vi "Write CRDS.vi"(8 "error in (no error)":errorcluster, 10 "CRDS":refnum<class "CRDS Data.lvclass">, 11 "Nicholas Data in":refnum<class "Nicholas Data.lvclass">) -> (0 "error out":errorcluster, 3 "Nicholas Data out":refnum<class "Nicholas Data.lvclass">)   [LabVIEW 2014, in "Nicholas Data.lvclass"]
uses:
  Nicholas Data.lvclass
  Reusable/CRDS/Data/Main/CRDS Data.lvclass
  Nicholas Data.lvclass/Nicholas Data.ctl
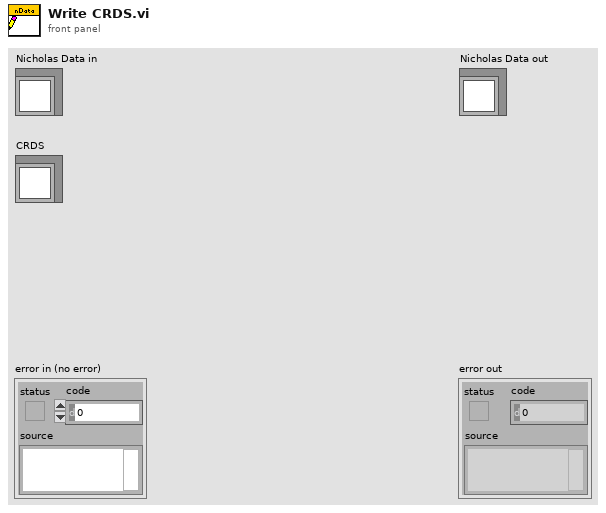
[diagram p1: front panel]
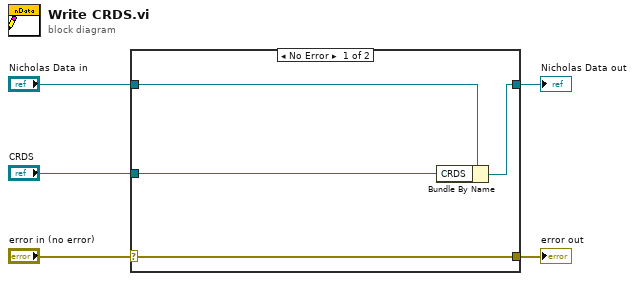
[diagram p0: block diagram]
diagram:
  n1 = case shown="No Error" "error in (no error)" {
    selector: "error in (no error)" -> [w9 w10]
    tunnel: [w9 w10] -> w4
    tunnel: [w7 w11] -> w2
    tunnel: "Nicholas Data in" -> [w8 w11]
    tunnel: "CRDS" -> [w6 _]
    frame No Error {
      n2 = Bundle By Name(cluster=w8, "CRDS"=w6) -> (w7:refnum<class "Nicholas Data.lvclass">)
    }
    frame Error {
    }
  }
  "error out" <- w4
  "Nicholas Data out" <- w2
